vi "Configure Frequency Period1.vi"(5 "Voltage Range (10: 10 V)":dbl(ring)=10.0 items=["0.1"=0.1, "1"=1.0, "10"=10.0, "100"=100.0, "1000"=1000.0], 6 "Auto Voltage Range (1: Enable)":i32(ring)=1 items=["Disable", "Enable", "Once"], 7 "AC Bandwidth (20: 20 Hz)":dbl(ring)=20.0 items=["3"=3.0, "20"=20.0, "200"=200.0], 8 "error in (no error)":errorcluster, 9 "Aperture Time (0.1: 0.1 s)":dbl(ring)=0.1 items=["0.01"=0.01, "0.1"=0.1, "1"=1.0], 10 "Frequency Period (0: Frequency)":i32(ring) items=["Frequency", "Period"], 11 "VISA resource name":refnum<visa-resource-name>) -> (0 "error out":errorcluster, 3 "VISA resource name out":refnum<visa-resource-name>)   [LabVIEW 2015, in "Agilent 3446X Series1.lvlib"]
doc: "Configures frequency and period measurements."
uses:
  Agilent 3446X Series1.lvlib
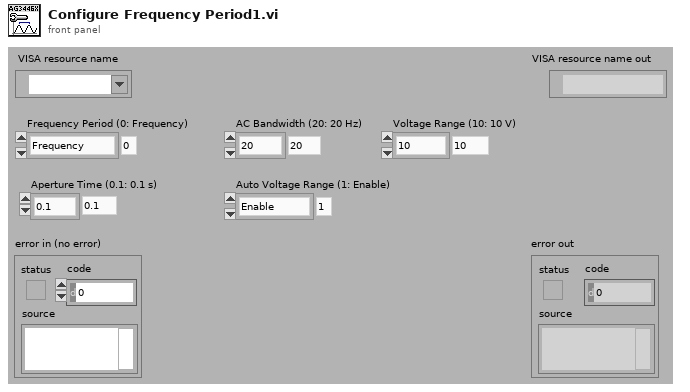
[diagram p1: front panel]
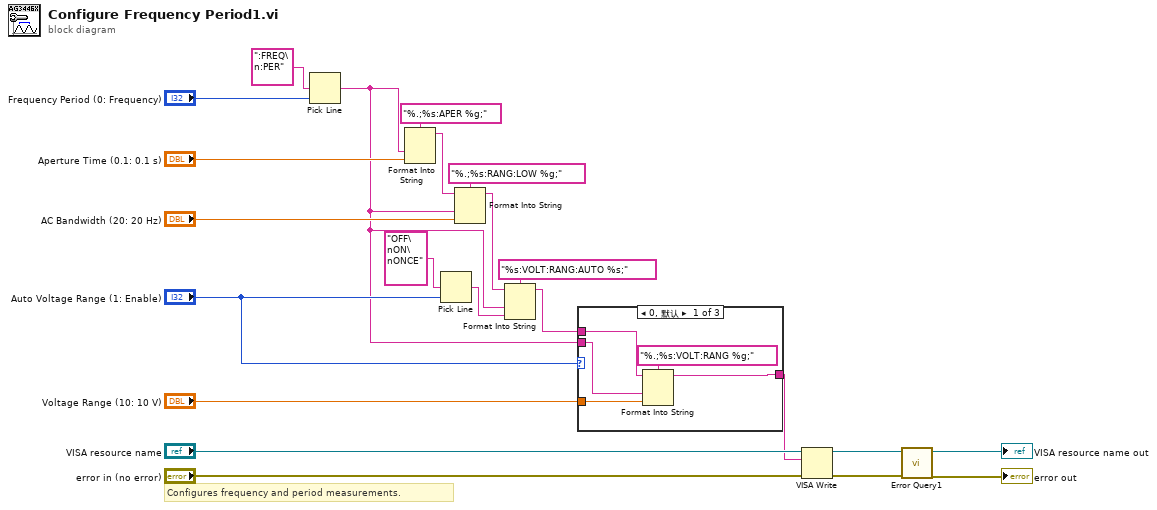
[diagram p0: block diagram]
diagram:
  # "Configures frequency and period measurements."
  n1 = Pick Line(multi-line string=":FREQ\n:PER", line index="Frequency Period (0: Frequency)") -> (output string=w3:string)  [unwired: 1 out]
  n2 = Format Into String(format string="%.;%s:APER %g;", w3, "Aperture Time (0.1: 0.1 s)") -> (resulting string=w18:string)  [unwired: 2 in, 1 out]
  n3 = Pick Line(multi-line string="OFF\nON\nONCE", line index="Auto Voltage Range (1: Enable)") -> (output string=w12:string)  [unwired: 1 out]
  n4 = Format Into String(format string="%.;%s:RANG:LOW %g;", initial string=w18, w3, "AC Bandwidth (20: 20 Hz)") -> (resulting string=w14:string)  [unwired: 1 in, 1 out]
  n5 = Format Into String(format string="%s:VOLT:RANG:AUTO %s;", initial string=w14, w3, w12) -> (resulting string=w2:string)  [unwired: 1 in, 1 out]
  n6 = case shown="0, 默认" "Auto Voltage Range (1: Enable)" {
    tunnel: "Voltage Range (10: 10 V)" -> [w26 _ _]
    tunnel: w3 -> [w25 _ _]
    tunnel: w2 -> [w24 w28 w29]
    tunnel: [w23 w28 w29] -> w1
    frame 0, Default {
      n7 = Format Into String(format string="%.;%s:VOLT:RANG %g;", initial string=w24, w25, w26) -> (resulting string=w23:string)  [unwired: 1 in, 1 out]
    }
    frame 1 {
    }
    frame 2 {
    }
  }
  n8 = VISA Write(VISA resource name="VISA resource name", write buffer=w1, error in (no error)="error in (no error)") -> (VISA resource name out=w9:refnum<visa-resource-name>, error out=w8:errorcluster)  [unwired: 1 out]
  n9 = call "Error Query1.vi"("error in (no error)"=w8, "VISA resource name"=w9) -> ("error out"=→"error out":errorcluster, "VISA resource name out"=→"VISA resource name out":refnum<visa-resource-name>)  [unwired: 8 out]
